vi "ExperimentSeries2_Init.vi"(0 "object in":refnum<class "ExperimentSeries2.lvclass">, 5 "error in (no error)":errorcluster) -> (14 "object out":refnum<class "ExperimentSeries2.lvclass">, 19 "error out":errorcluster)   [LabVIEW 2021, in "ExperimentSeries2.lvclass"]
uses:
  ExperimentSeries2.lvclass
  Experiment2_class/Experiment2.lvclass
  ExperimentSeries2.lvclass/ExperimentSeries2.ctl
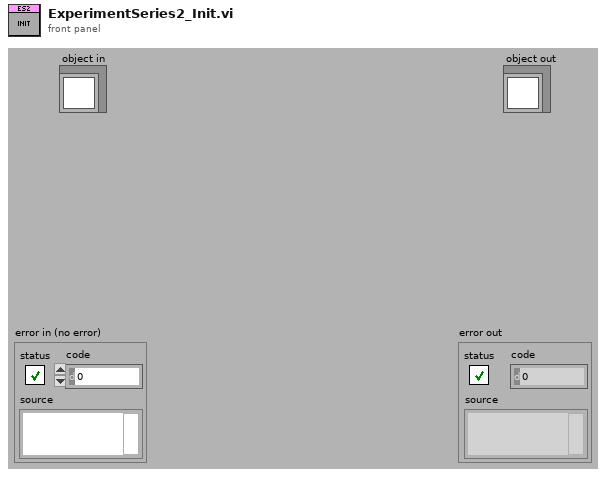
[diagram p1: front panel]
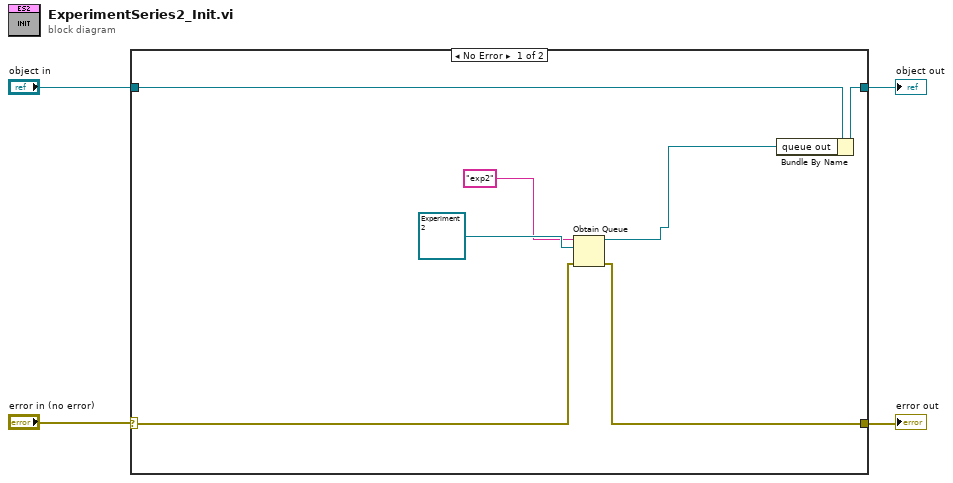
[diagram p0: block diagram]
diagram:
  n1 = case shown="No Error" "error in (no error)" {
    selector: "error in (no error)" -> [w9 w12]
    tunnel: "object in" -> [w11 w13]
    tunnel: [w10 w13] -> w3
    tunnel: [w8 w12] -> w1
    frame No Error {
      n2 = Obtain Queue(name (unnamed)="exp2", element data type=refnum<class "Experiment2.lvclass"> refnum ("Experiment2"), error in (no error)=w9) -> (queue out=w6:refnum<queue>, error out=w8:errorcluster)  [unwired: 2 in, 1 out]
      n3 = Bundle By Name(cluster=w11, "queue out"=w6) -> (w10:refnum<class "ExperimentSeries2.lvclass">)
    }
    frame Error {
    }
  }
  "object out" <- w3
  "error out" <- w1
